vi "MSE310Project.vi"() -> ()   [LabVIEW 2016]
uses:
  MSE310 Project Control.ctl
  <vilib>/DAQmx/read.llb/DAQmx Read (Digital Bool 1Line 1Point).vi
  <vilib>/DAQmx/write.llb/DAQmx Write (Digital Bool 1Line 1Point).vi
  <vilib>/DAQmx/create/channels.llb/DAQmx Create Channel (DO-Digital Output).vi
  <vilib>/DAQmx/create/channels.llb/DAQmx Create Channel (DI-Digital Input).vi
  <vilib>/DAQmx/miscellaneous.llb/DAQmx Fill In Error Info.vi
panel:
  in  "stop 2":bool
  out "TIMER_FLAG":bool
  out "KICK_COUNT_BOOL-1":bool
  out "KICK_COUNT_BOOL":bool
  out "TOP_PUSH-1":bool
  out "HOP_LIT_SENS-1":bool
  out "KICK_FLAG-1":bool
  out "KICK_FLAG":bool
  out "TOTAL_ASM":u16
  out "HOPPER":bool
  out "KICK_COUNT":u16
  out "HOP_LIT_SENS":bool
  out "TOP_PUSH":bool
  out "RUNNING":bool
  out "START":bool
  out "TOP_LIT_SENS":bool
  out "TOP_MAT_SENS":bool
  out "STOP":T1
  in  "stop":bool
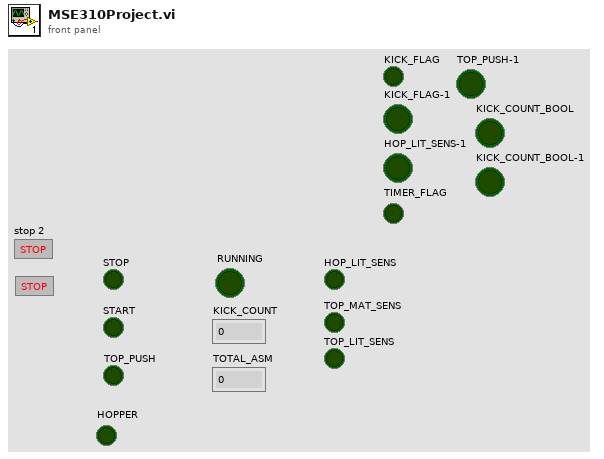
[diagram p1: front panel]
types:
  T1 = typedef "MSE310 Project Control.ctl" = bool
  T2 = cluster{"task out":refnum<k21>, "error out":errorcluster, "task out":refnum<k21>, "error out":errorcluster, "task out":refnum<k21>, "error out":errorcluster, "task out":refnum<k21>, "error out":errorcluster}
  T3 = cluster{"task out":refnum<k21>, "error out":errorcluster, "task out":refnum<k21>, "error out":errorcluster, "task out":refnum<k21>, "error out":errorcluster, "task out":refnum<k21>, "error out":errorcluster, "task out":refnum<k21>, "error out":errorcluster}
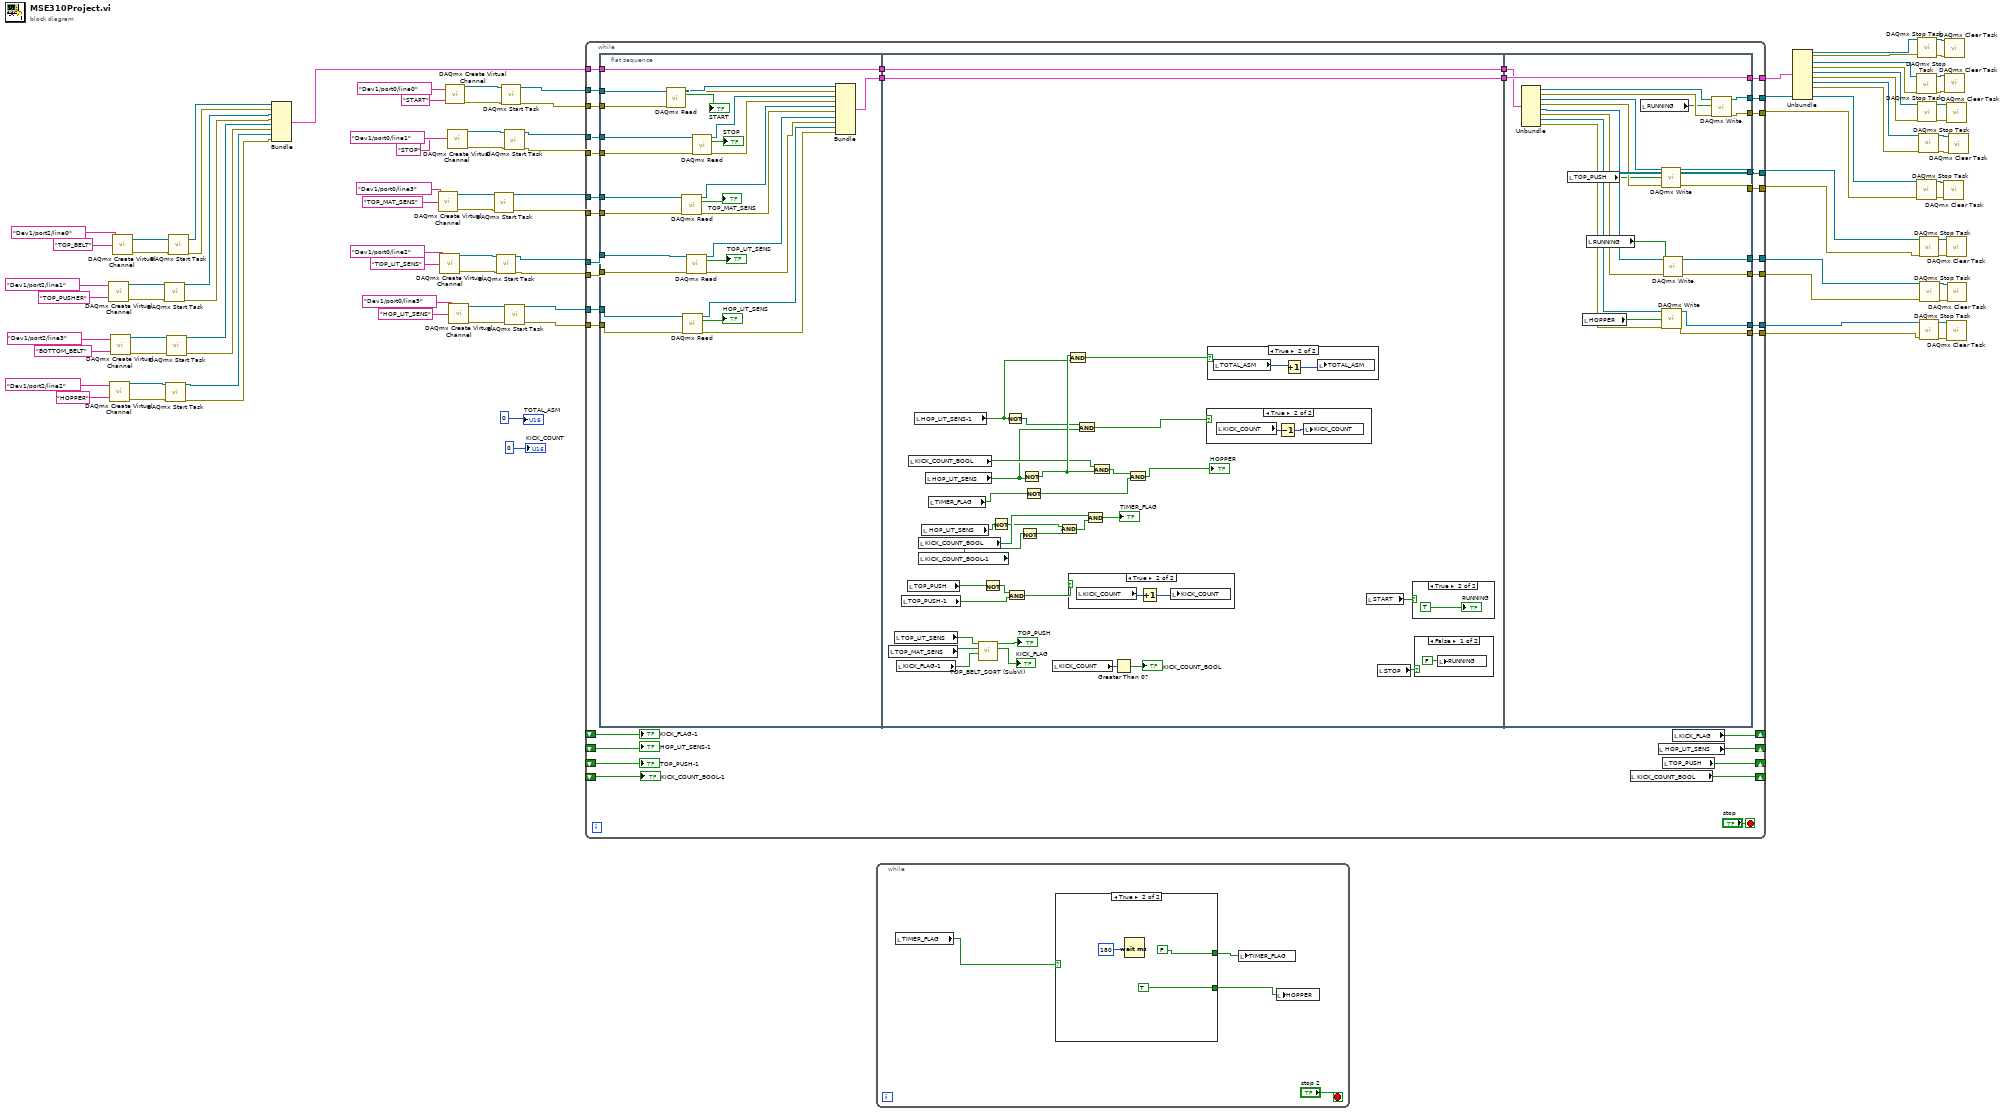
[diagram p0: block diagram]
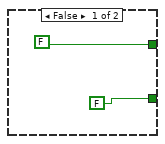
[diagram p2: hidden frame]
diagram:
  n1 = call-poly <vilib>:"DAQmx Create Virtual Channel.vi"("lines"=tag "Dev1/port2/line1", "name to assign"="TOP_PUSHER") -> ("task out"=w85:refnum<k21>, "error out"=w86:errorcluster)  [unwired: 12 in]
  n2 = call-poly <vilib>:"DAQmx Create Virtual Channel.vi"("lines"=tag "Dev1/port2/line2", "name to assign"="HOPPER") -> ("task out"=w10:refnum<k21>, "error out"=w11:errorcluster)  [unwired: 12 in]
  n3 = call-poly <vilib>:"DAQmx Create Virtual Channel.vi"("lines"=tag "Dev1/port2/line3", "name to assign"="BOTTOM_BELT") -> ("task out"=w32:refnum<k21>, "error out"=w33:errorcluster)  [unwired: 12 in]
  n4 = call-poly <vilib>:"DAQmx Create Virtual Channel.vi"("lines"=tag "Dev1/port2/line0", "name to assign"="TOP_BELT") -> ("task out"=w77:refnum<k21>, "error out"=w78:errorcluster)  [unwired: 12 in]
  n5 = call <vilib>:"DAQmx Start Task.vi"("task/channels in"=w85, "error in"=w86) -> ("task out"=w45:refnum<k21>, "error out"=w44:errorcluster)  [unwired: 12 in]
  n6 = call <vilib>:"DAQmx Start Task.vi"("task/channels in"=w10, "error in"=w11) -> ("task out"=w8:refnum<k21>, "error out"=w7:errorcluster)  [unwired: 12 in]
  n7 = call <vilib>:"DAQmx Start Task.vi"("task/channels in"=w32, "error in"=w33) -> ("task out"=w31:refnum<k21>, "error out"=w30:errorcluster)  [unwired: 12 in]
  n8 = call <vilib>:"DAQmx Start Task.vi"("task/channels in"=w77, "error in"=w78) -> ("task out"=w47:refnum<k21>, "error out"=w46:errorcluster)  [unwired: 12 in]
  n9 = Bundle("task out"=w47, "error out"=w46, "task out"=w45, "error out"=w44, "task out"=w31, "error out"=w30, "task out"=w8, "error out"=w7) -> (w43:T2)  [unwired: 1 in]
  n10 = call-poly <vilib>:"DAQmx Create Virtual Channel.vi"("lines"=tag "Dev1/port0/line3", "name to assign"="TOP_MAT_SENS") -> ("task out"=w82:refnum<k21>, "error out"=w83:errorcluster)  [unwired: 12 in]
  n11 = call-poly <vilib>:"DAQmx Create Virtual Channel.vi"("lines"=tag "Dev1/port0/line2", "name to assign"="TOP_LIT_SENS") -> ("task out"=w88:refnum<k21>, "error out"=w89:errorcluster)  [unwired: 12 in]
  n12 = call-poly <vilib>:"DAQmx Create Virtual Channel.vi"("lines"=tag "Dev1/port0/line0", "name to assign"="START") -> ("task out"=w73:refnum<k21>, "error out"=w74:errorcluster)  [unwired: 12 in]
  n13 = call-poly <vilib>:"DAQmx Create Virtual Channel.vi"("lines"=tag "Dev1/port0/line1", "name to assign"="STOP") -> ("task out"=w75:refnum<k21>, "error out"=w76:errorcluster)  [unwired: 12 in]
  n14 = call-poly <vilib>:"DAQmx Create Virtual Channel.vi"("lines"=tag "Dev1/port0/line5", "name to assign"="HOP_LIT_SENS") -> ("task out"=w16:refnum<k21>, "error out"=w17:errorcluster)  [unwired: 12 in]
  n15 = call <vilib>:"DAQmx Start Task.vi"("task/channels in"=w82, "error in"=w83) -> ("task out"=w70:refnum<k21>, "error out"=w69:errorcluster)  [unwired: 12 in]
  n16 = call <vilib>:"DAQmx Start Task.vi"("task/channels in"=w88, "error in"=w89) -> ("task out"=w68:refnum<k21>, "error out"=w67:errorcluster)  [unwired: 12 in]
  n17 = call <vilib>:"DAQmx Start Task.vi"("task/channels in"=w73, "error in"=w74) -> ("task out"=w66:refnum<k21>, "error out"=w65:errorcluster)  [unwired: 12 in]
  n18 = call <vilib>:"DAQmx Start Task.vi"("task/channels in"=w75, "error in"=w76) -> ("task out"=w72:refnum<k21>, "error out"=w71:errorcluster)  [unwired: 12 in]
  n19 = call <vilib>:"DAQmx Start Task.vi"("task/channels in"=w16, "error in"=w17) -> ("task out"=w14:refnum<k21>, "error out"=w13:errorcluster)  [unwired: 12 in]
  n20 = while {
    tunnel: w72 -> [w122]
    tunnel: w71 -> [w121]
    tunnel: w70 -> [w120]
    tunnel: w69 -> [w119]
    tunnel: w68 -> [w118]
    tunnel: w67 -> [w117]
    tunnel: w66 -> [w116]
    tunnel: w65 -> [w115]
    tunnel: [w114] -> w64
    tunnel: w43 -> [w109]
    tunnel: [w108] -> w41
    tunnel: [w107] -> w40
    tunnel: [w106] -> w36
    tunnel: [w105] -> w35
    tunnel: [w104] -> w27
    tunnel: [w103] -> w26
    shift-right: [w98] -> _
    shift-left: _ -> [w97]
    tunnel: w14 -> [w102]
    tunnel: w13 -> [w101]
    tunnel: [w100] -> w4
    tunnel: [w99] -> w3
    shift-right: [w96] -> _
    shift-left: _ -> [w95]
    shift-right: [w94] -> _
    shift-left: _ -> [w93]
    shift-right: [w92] -> _
    shift-left: _ -> [w91]
    stop <- "stop" stop-if-true
    n21 = flat-sequence {
      tunnel: w122 -> [w150]
      tunnel: w121 -> [w149]
      tunnel: w120 -> [w147]
      tunnel: w119 -> [w146]
      tunnel: w118 -> [w145]
      tunnel: w117 -> [w144]
      tunnel: w116 -> [w141]
      tunnel: w115 -> [w140]
      tunnel: [w130] -> w112
      tunnel: [w129] -> w110
      tunnel: w109 -> [w129]
      tunnel: w102 -> [w127]
      tunnel: w101 -> [w126]
      tunnel: [w183] -> w113
      tunnel: w112 -> [w183]
      tunnel: [w182] -> w111
      tunnel: w110 -> [w182]
      tunnel: [w213] -> w114
      tunnel: w113 -> [w213]
      tunnel: w111 -> [w212]
      tunnel: [w207] -> w108
      tunnel: [w206] -> w107
      tunnel: [w205] -> w106
      tunnel: [w204] -> w105
      tunnel: [w201] -> w104
      tunnel: [w200] -> w103
      tunnel: [w194] -> w100
      tunnel: [w193] -> w99
      frame #0 {
        n22 = call-poly <vilib>:"DAQmx Read.vi"("task/channels in"=w141, "error in"=w140) -> ("task out"=w138:refnum<k21>, "data"=→"START":bool, "error out"=w137:errorcluster)  [unwired: 11 in]
        n23 = call-poly <vilib>:"DAQmx Read.vi"("task/channels in"=w147, "error in"=w146) -> ("task out"=w134:refnum<k21>, "data"=→"TOP_MAT_SENS":bool, "error out"=w133:errorcluster)  [unwired: 11 in]
        n24 = call-poly <vilib>:"DAQmx Read.vi"("task/channels in"=w127, "error in"=w126) -> ("task out"=w125:refnum<k21>, "data"=→"HOP_LIT_SENS":bool, "error out"=w124:errorcluster)  [unwired: 11 in]
        n25 = call-poly <vilib>:"DAQmx Read.vi"("task/channels in"=w145, "error in"=w144) -> ("task out"=w132:refnum<k21>, "data"=→"TOP_LIT_SENS":bool, "error out"=w131:errorcluster)  [unwired: 11 in]
        n26 = call-poly <vilib>:"DAQmx Read.vi"("task/channels in"=w150, "error in"=w149) -> ("task out"=w136:refnum<k21>, "data"=→"STOP":bool, "error out"=w135:errorcluster)  [unwired: 11 in]
        n27 = Bundle("task out"=w138, "error out"=w137, "task out"=w136, "error out"=w135, "task out"=w134, "error out"=w133, "task out"=w132, "error out"=w131, "task out"=w125, "error out"=w124) -> (w130:T3)  [unwired: 1 in]
      }
      frame #1 {
        n28 = local read "TOP_MAT_SENS"() -> (w169:bool)
        n29 = local read "TOP_LIT_SENS"() -> (w171:bool)
        n30 = local read "KICK_FLAG-1"() -> (w172:bool)
        n31 = local read "TOP_PUSH-1"() -> (w167:bool)
        n32 = local read "TOP_PUSH"() -> (w166:bool)
        n33 = local read "KICK_COUNT_BOOL"() -> (w165:bool)
        n34 = local read "HOP_LIT_SENS-1"() -> (w162:bool)
        n35 = local read "KICK_COUNT_BOOL"() -> (w161:bool)
        n36 = local read "KICK_COUNT_BOOL-1"() -> (w159:bool)
        n37 = local read "HOP_LIT_SENS"() -> (w157:bool)
        n38 = local read "HOP_LIT_SENS"() -> (w164:bool)
        n39 = local read "TIMER_FLAG"() -> (w153:bool)
        n40 = call "TOP_BELT_SORT (SubVI).vi"("KICK_FLAG-1"=w172, "TOP_MAT_SENS"=w169, "TOP_LIT_SENS"=w171) -> ("Boolean"=→"KICK_FLAG":bool, "Boolean 2"=→"TOP_PUSH":bool)  [unwired: 7 in]
        n41 = Not(x=w166) -> (.not. x?=w174:bool)
        n42 = Not(x=w157) -> (.not. x?=w156:bool)
        n43 = Not(x=w162) -> (.not. x?=w163:bool)
        n44 = And(x=w174, y=w167) -> (x .and. y?=w175:bool)
        n45 = Not(x=w159) -> (.not. x?=w158:bool)
        n46 = Not(x=w164) -> (.not. x?=w176:bool)
        n47 = Not(x=w153) -> (.not. x?=w152:bool)
        n48 = local read "KICK_COUNT"() -> (w179:u16)
        n49 = And(x=w156, y=w158) -> (x .and. y?=w160:bool)
        n50 = And(x=w176, y=w162) -> (x .and. y?=w177:bool)
        n51 = case shown="True" w175 {
          frame False {
          }
          frame True {
            n52 = local read "KICK_COUNT"() -> (w189:u16)
            n53 = Increment(x=w189) -> (x+1=w188:u16)
            n54 = local write "KICK_COUNT"(w188) -> ()
          }
        }
        n55 = And(x=w163, y=w164) -> (x .and. y?=w178:bool)
        n56 = And(x=w161, y=w160) -> (x .and. y?=→"TIMER_FLAG":bool)
        n57 = And(x=w165, y=w176) -> (x .and. y?=w154:bool)
        n58 = Greater Than 0?(x=w179) -> (x > 0?=→"KICK_COUNT_BOOL":bool)
        n59 = And(x=w154, y=w152) -> (x .and. y?=→"HOPPER":bool)
        n60 = case shown="True" w178 {
          frame False {
          }
          frame True {
            n61 = local read "KICK_COUNT"() -> (w187:u16)
            n62 = Decrement(x=w187) -> (x-1=w186:u16)
            n63 = local write "KICK_COUNT"(w186) -> ()
          }
        }
        n64 = case shown="True" w177 {
          frame False {
          }
          frame True {
            n65 = local read "TOTAL_ASM"() -> (w185:u16)
            n66 = Increment(x=w185) -> (x+1=w184:u16)
            n67 = local write "TOTAL_ASM"(w184) -> ()
          }
        }
        n68 = local read "START"() -> (w180:bool)
        n69 = local read "STOP"() -> (w181:T1)
        n70 = case shown="True" w180 {
          frame False {
          }
          frame True {
            "RUNNING" <- TRUE ("RUNNING")
          }
        }
        n71 = case shown="False" w181 {
          frame False {
            n72 = local write "RUNNING"(FALSE ("RUNNING")) -> ()
          }
          frame True {
          }
        }
      }
      frame #2 {
        n73 = Unbundle(w212) -> ("task out"=w211:refnum<k21>, "error out"=w210:errorcluster, "task out"=w209:refnum<k21>, "error out"=w208:errorcluster, "task out"=w203:refnum<k21>, "error out"=w202:errorcluster, "task out"=w196:refnum<k21>, "error out"=w195:errorcluster)
        n74 = local read "TOP_PUSH"() -> (w197:bool)
        n75 = local read "HOPPER"() -> (w192:bool)
        n76 = local read "RUNNING"() -> (w198:bool)
        n77 = local read "RUNNING"() -> (w199:bool)
        n78 = call-poly <vilib>:"DAQmx Write.vi"("task/channels in"=w209, "data"=w197, "error in"=w208) -> ("task out"=w205:refnum<k21>, "error out"=w204:errorcluster)  [unwired: 10 in, 1 out]
        n79 = call-poly <vilib>:"DAQmx Write.vi"("task/channels in"=w196, "data"=w192, "error in"=w195) -> ("task out"=w194:refnum<k21>, "error out"=w193:errorcluster)  [unwired: 10 in, 1 out]
        n80 = call-poly <vilib>:"DAQmx Write.vi"("task/channels in"=w203, "data"=w198, "error in"=w202) -> ("task out"=w201:refnum<k21>, "error out"=w200:errorcluster)  [unwired: 10 in, 1 out]
        n81 = call-poly <vilib>:"DAQmx Write.vi"("task/channels in"=w211, "data"=w199, "error in"=w210) -> ("task out"=w207:refnum<k21>, "error out"=w206:errorcluster)  [unwired: 10 in, 1 out]
      }
    }
    n82 = local read "KICK_COUNT_BOOL"() -> (w92:bool)
    n83 = local read "HOP_LIT_SENS"() -> (w96:bool)
    n84 = local read "TOP_PUSH"() -> (w94:bool)
    n85 = local read "KICK_FLAG"() -> (w98:bool)
    "KICK_FLAG-1" <- w97
    "HOP_LIT_SENS-1" <- w95
    "TOP_PUSH-1" <- w93
    "KICK_COUNT_BOOL-1" <- w91
  }
  n86 = while {
    stop <- "stop 2" stop-if-true
    n87 = local read "TIMER_FLAG"() -> (w215:bool)
    n88 = case shown="True" w215 {
      tunnel: [FALSE TRUE] -> w217
      tunnel: [FALSE FALSE] -> w216
      frame False {
      }
      frame True {
        n89 = Wait (ms)(milliseconds to wait=180) -> ()  [unwired: 1 out]
      }
    }
    n90 = local write "TIMER_FLAG"(w216) -> ()
    n91 = local write "HOPPER"(w217) -> ()
  }
  n92 = Unbundle(w64) -> ("task out"=w61:refnum<k21>, "error out"=w60:errorcluster, "task out"=w57:refnum<k21>, "error out"=w56:errorcluster, "task out"=w51:refnum<k21>, "error out"=w50:errorcluster, "task out"=w49:refnum<k21>, "error out"=w48:errorcluster)  [unwired: 2 out]
  n93 = call <vilib>:"DAQmx Stop Task.vi"("task/channels in"=w57, "error in"=w56) -> ("task out"=w59:refnum<k21>, "error out"=w58:errorcluster)  [unwired: 12 in]
  n94 = call <vilib>:"DAQmx Stop Task.vi"("task/channels in"=w41, "error in"=w40) -> ("task out"=w42:refnum<k21>, "error out"=w38:errorcluster)  [unwired: 12 in]
  n95 = call <vilib>:"DAQmx Stop Task.vi"("task/channels in"=w61, "error in"=w60) -> ("task out"=w63:refnum<k21>, "error out"=w62:errorcluster)  [unwired: 12 in]
  n96 = call <vilib>:"DAQmx Stop Task.vi"("task/channels in"=w51, "error in"=w50) -> ("task out"=w55:refnum<k21>, "error out"=w54:errorcluster)  [unwired: 12 in]
  n97 = call <vilib>:"DAQmx Stop Task.vi"("task/channels in"=w49, "error in"=w48) -> ("task out"=w53:refnum<k21>, "error out"=w52:errorcluster)  [unwired: 12 in]
  n98 = call <vilib>:"DAQmx Stop Task.vi"("task/channels in"=w36, "error in"=w35) -> ("task out"=w39:refnum<k21>, "error out"=w37:errorcluster)  [unwired: 12 in]
  n99 = call <vilib>:"DAQmx Stop Task.vi"("task/channels in"=w4, "error in"=w3) -> ("task out"=w6:refnum<k21>, "error out"=w5:errorcluster)  [unwired: 12 in]
  n100 = call <vilib>:"DAQmx Stop Task.vi"("task/channels in"=w27, "error in"=w26) -> ("task out"=w29:refnum<k21>, "error out"=w28:errorcluster)  [unwired: 12 in]
  n101 = call <vilib>:"DAQmx Clear Task.vi"("task in"=w42, "error in"=w38) -> ()  [unwired: 13 in, 1 out]
  n102 = call <vilib>:"DAQmx Clear Task.vi"("task in"=w63, "error in"=w62) -> ()  [unwired: 13 in, 1 out]
  n103 = call <vilib>:"DAQmx Clear Task.vi"("task in"=w59, "error in"=w58) -> ()  [unwired: 13 in, 1 out]
  n104 = call <vilib>:"DAQmx Clear Task.vi"("task in"=w55, "error in"=w54) -> ()  [unwired: 13 in, 1 out]
  n105 = call <vilib>:"DAQmx Clear Task.vi"("task in"=w39, "error in"=w37) -> ()  [unwired: 13 in, 1 out]
  n106 = call <vilib>:"DAQmx Clear Task.vi"("task in"=w6, "error in"=w5) -> ()  [unwired: 13 in, 1 out]
  n107 = call <vilib>:"DAQmx Clear Task.vi"("task in"=w29, "error in"=w28) -> ()  [unwired: 13 in, 1 out]
  n108 = call <vilib>:"DAQmx Clear Task.vi"("task in"=w53, "error in"=w52) -> ()  [unwired: 13 in, 1 out]
  "TOTAL_ASM" <- u16 0 ("TOTAL_ASM")
  "KICK_COUNT" <- u16 0 ("KICK_COUNT")
